vi "DriveEngine.vi"(6 "RTrigger_Axis":dbl, 7 "GyroData":T1, 9 "LTrigger_Axis":dbl, 10 "LY_Axis":dbl, 11 "LX_Axis":dbl) -> (0 "error out":errorcluster, 1 "RotationCmd":dbl, 2 "Y_AxisCmd":dbl, 3 "X_AxisCmd":dbl, 5 "Motor Values":dbl[](array[numeric]))   [LabVIEW 2017]
uses:
  Support Code/Gyro/Gyro_TypeDef.ctl
  <vilib>/Rock Robotics/WPI/Utilities/WPI_GetSetVariantRefNum.vi
  <vilib>/Rock Robotics/WPI/RobotDrive/WPI_RobotDriveMecanumDrive_Cartesian.vi
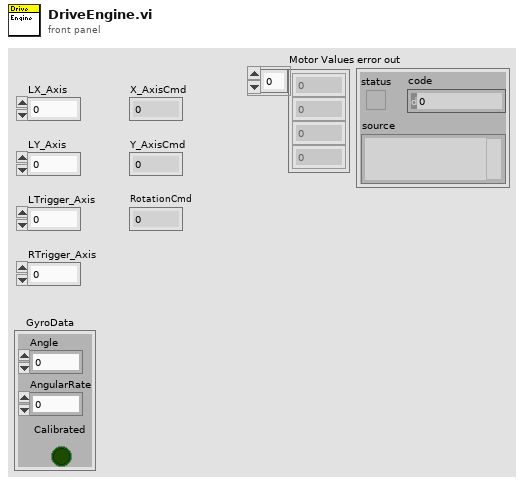
[diagram p1: front panel]
types:
  T1 = typedef "Gyro_TypeDef.ctl" = cluster{"Angle":dbl, "AngularRate":dbl, "Calibrated":bool}
  T2 = typedef "WPI_RobotDriveDevRef.ctl" = cluster{"DevStatus":errorcluster, "Motors[]":T3[], "Square Inputs":bool, "Max Output":dbl}
  T3 = typedef "WPI_MotorControlDeviceRef.ctl" = cluster{"DeviceStatus":errorcluster, "Type":T4, "PWM":cluster{"PWM Channel":T5, "DeadBand":T6}, "CAN":cluster{"Device Number":u8, "SetOutput VI Ref":variant, "GetOutput VI Ref":variant, "Enable VI Ref":variant, "Disable VI Ref":variant, "Data":variant}, "Invert":bool, "DIO PWM":cluster{"PWM \"Enable\" Channel":T5, "DIOChannel":T7, "PWM Rate":dbl}}
  T4 = typedef "WPI_MotorControlType.ctl" = enum16{"PWM", "CAN", "DIO PWM"}
  T5 = typedef "FPGA_DIOPWMChannel.ctl" = enum8{"PWM 0", "PWM 1", "PWM 2", "PWM 3", "PWM 4", "PWM 5", "PWM 6", "PWM 7", "PWM 8", "PWM 9", "PWM MXP 0", "PWM MXP 1", "PWM MXP 2", "PWM MXP 3", "PWM MXP 4", "PWM MXP 5", "PWM MXP 6", "PWM MXP 7", "PWM MXP 8", "PWM MXP 9", "Invalid"}
  T6 = typedef "WPI_PWMDeadband.ctl" = cluster{"Name":string, "maxPositivePwm":i32, "minPositivePwm":i32, "centerPwm":i32, "maxNegativePwm":i32, "minNegativePwm":i32, "angularRange":u16}
  T7 = typedef "FPGA_DIOChannel.ctl" = enum8{"DIO 0", "DIO 1", "DIO 2", "DIO 3", "DIO 4", "DIO 5", "DIO 6", "DIO 7", "DIO 8", "DIO 9", "DIO MXP 0", "DIO MXP 1", "DIO MXP 2", "DIO MXP 3", "DIO MXP 4", "DIO MXP 5", "DIO MXP 6", "DIO MXP 7", "DIO MXP 8", "DIO MXP 9", "DIO MXP 10", "DIO MXP 11", "DIO MXP 12", "DIO MXP 13", "DIO MXP 14", "DIO MXP 15", "SPI Port CS1", "SPI Port CS2", "SPI Port CS3", "SPI Port MISO", "SPI Port MOSI", "Invalid"}
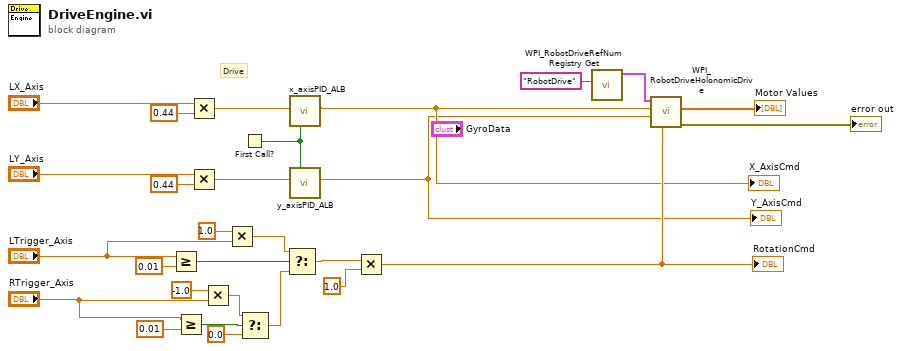
[diagram p0: block diagram]
diagram:
  # "Drive"
  n1 = Greater Or Equal?(x="LTrigger_Axis", y=0.01) -> (x >= y?=w17:bool)
  n2 = Greater Or Equal?(x="RTrigger_Axis", y=0.01) -> (x >= y?=w12:bool)
  n3 = Multiply(x="LX_Axis", y=0.44) -> (x*y=w7:dbl)
  n4 = Multiply(x="LY_Axis", y=0.44) -> (x*y=w5:dbl)
  n5 = Multiply(x=-1.0, y="RTrigger_Axis") -> (x*y=w13:dbl)
  n6 = Multiply(x=1.0, y="LTrigger_Axis") -> (x*y=w21:dbl)
  n7 = First Call?() -> (First Call?: T/F=w3:bool)
  n8 = Select(t=w13, s=w12, f=0.0) -> (s? t:f=w18:dbl)
  n9 = Select(t=w21, s=w17, f=w18) -> (s? t:f=w22:dbl)
  n10 = call "x_axisPID_ALB.vi"("First Call?: T/F"=w3, "x axis"=w7) -> ("x axis out"=w6:dbl)  [unwired: 9 in]
  "X_AxisCmd" <- w6
  n11 = call "y_axisPID_ALB.vi"("First Call?: T/F"=w3, "y axis"=w5) -> ("y axis out"=w4:dbl)  [unwired: 9 in]
  "Y_AxisCmd" <- w4
  n12 = Multiply(x=w22, y=1.0) -> (x*y=w28:dbl)
  "RotationCmd" <- w28
  n13 = call <vilib>:"WPI_RobotDriveRefNum Registry Get.vi"("refnum name"="RobotDrive") -> ("RobotDriveDevRef"=w9:T2)  [unwired: 9 in, 1 out]
  n14 = call-poly <vilib>:"WPI_RobotDriveHolonomicDrive.vi"("Rotation"=w28, "Y"=w4, "X"=w6, "RobotDriveDevRef"=w9) -> ("error out"=→"error out":errorcluster, "Motor Values"=→"Motor Values":dbl[])  [unwired: 5 in, 1 out]
